vi "isMotorOn.vi"(3 "Device":refnum<k24>) -> (0 "isConnected":bool, 1 "Device out":refnum<k24>)   [LabVIEW 2021]
doc: "André Romero - 2017\nandretec@ifsc.usp.br"
uses:
  C:/user-Lab/AndreTec/GITs/andretec/Thorlabs-Vector-Move/kinesisTec/Kinesis/Thorlabs.MotionControl.TCube.DCServoCLI.dll
  Kinesis/Thorlabs.MotionControl.TCube.DCServoCLI.dll
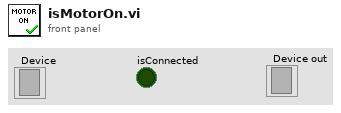
[diagram p1: front panel]
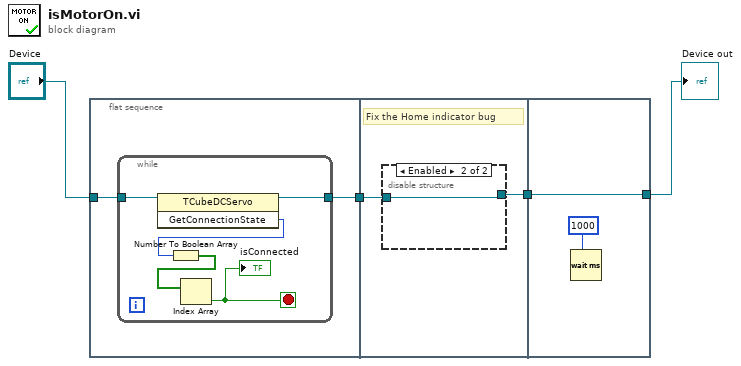
[diagram p0: block diagram]
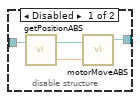
[diagram p2: hidden frame]
diagram:
  n1 = flat-sequence {
    tunnel: "Device" -> [w6]
    tunnel: [w5] -> w3
    tunnel: w3 -> [w13]
    tunnel: [w12] -> w1
    tunnel: [w19] -> w2
    tunnel: w1 -> [w19]
    frame #0 {
      n2 = while {
        tunnel: w6 -> [w11]
        tunnel: [w7] -> w5
        stop <- w8 stop-if-true
        n3 = invoke class="TCubeDCServo" method="GetConnectionState"(reference=w11) -> (reference out=w7:refnum<k24>, "GetConnectionState"=w10:i32)  [unwired: 2 in, 1 out]
        n4 = Number To Boolean Array(number=w10) -> (Boolean array=w9:bool[])
        n5 = Index Array(array=w9) -> (element=w8:bool)  [unwired: 1 in]
        "isConnected" <- w8
      }
    }
    frame #1 {
      # "Fix the Home indicator bug"
      n6 = disable-structure shown="Enabled" {
        disable-tunnel: w13 -> [w17 w18]
        disable-tunnel: [w14 w18] -> w12
        frame Disabled {
          n7 = call "getPositionABS.vi"("Device"=w17) -> ("GetPOS"=w16:dbl, "Device out"=w15:refnum<k24>)  [unwired: 1 in]
          n8 = call "motorMoveABS.vi"("position"=w16, "Device in"=w15) -> ("Device out"=w14:refnum<k24>)  [unwired: 3 in]
        }
        frame Enabled {
        }
      }
    }
    frame #2 {
      n9 = Wait (ms)(milliseconds to wait=u32 1000) -> ()  [unwired: 1 out]
    }
  }
  "Device out" <- w2
